vi "9by9GridOfSpots.vi"(9 "GridSpotsNoiseAmp":dbl, 10 "Grid Size Y":i32, 11 "Grid Size x":i32) -> (3 "Spot Params":T1 {"Z" format="%_4g"; "Y" format="%_4g"; "X" format="%_4g"; "Phase" format="%_4g"; "Intensity" format="%_4g"})   [LabVIEW 2020]
uses:
  _controls/Spot Params.ctl
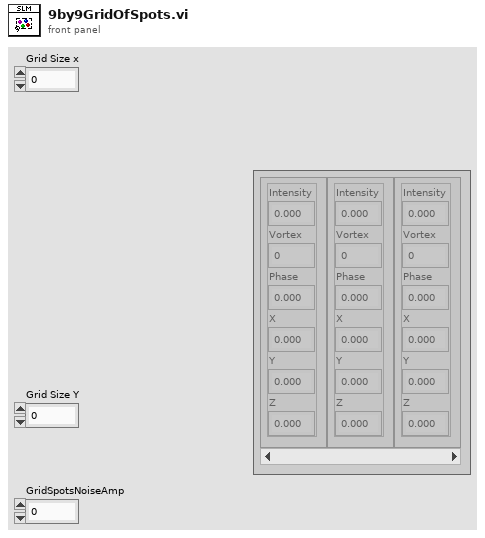
[diagram p1: front panel]
types:
  T1 = typedef "Spot Params.ctl" = cluster{"Intensity":dbl, "Vortex":dbl, "Phase":dbl, "X":dbl, "Y":dbl, "Z":dbl}[]
  T2 = cluster{"Intensity":dbl, "Vortex":dbl, "Phase":dbl, "X":dbl, "Y":dbl, "Z":dbl}
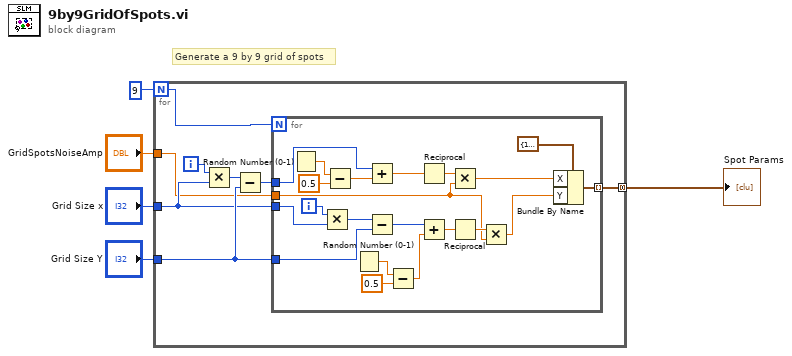
[diagram p0: block diagram]
diagram:
  # "Generate a 9 by 9 grid of spots"
  n1 = for {
    N: 9 -> [w13]
    tunnel: [w11] -> w1 mode=concatenating
    tunnel: "Grid Size Y" -> [w10]
    tunnel: "Grid Size x" -> [w7]
    tunnel: "GridSpotsNoiseAmp" -> [w6]
    i -> [w9]
    n2 = Multiply(x=w9, y=w7) -> (x*y=w8:i32)
    n3 = Subtract(x=w8, y=w10) -> (x-y=w12:i32)
    n4 = for {
      N: w13 -> [_]
      tunnel: w12 -> [w26]
      tunnel: [w22] -> w11 mode=indexing
      tunnel: w10 -> [w33]
      tunnel: w7 -> [w31]
      tunnel: w6 -> [w14]
      i -> [w32]
      n5 = Random Number (0-1)() -> (number: 0 to 1=w29:dbl)
      n6 = Multiply(x=w32, y=w31) -> (x*y=w30:i32)
      n7 = Subtract(x=w29, y=0.5) -> (x-y=w27:dbl)
      n8 = Random Number (0-1)() -> (number: 0 to 1=w15:dbl)
      n9 = Add(x=w26, y=w27) -> (x+y=w20:dbl)
      n10 = Subtract(x=w30, y=w33) -> (x-y=w23:i32)
      n11 = Subtract(x=w15, y=0.5) -> (x-y=w24:dbl)
      n12 = Reciprocal(x=w20) -> (1/x=w19:dbl)
      n13 = Add(x=w23, y=w24) -> (x+y=w21:dbl)
      n14 = Multiply(x=w19, y=w14) -> (x*y=w17:dbl)
      n15 = Reciprocal(x=w21) -> (1/x=w18:dbl)
      n16 = Multiply(x=w18, y=w14) -> (x*y=w16:dbl)
      n17 = Bundle By Name(cluster=T2 {"Intensity"=1.0, "Vortex"=0.0, "Phase"=0.0, "X"=0.0, "Y"=0.0, "Z"=0.0} ("Spot Settings"), "X"=w17, "Y"=w16) -> (w22:T2)
    }
  }
  "Spot Params" <- w1
